vi "TDMS文件浏览.vi"() -> ()   [LabVIEW 2010]
doc: "Writes channels of data to different groups in the TDMS file format."
panel:
  in  "file path":path caption="文件路径"
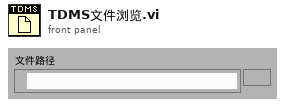
[diagram p1: front panel]
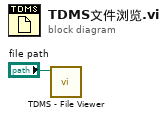
[diagram p0: block diagram]
diagram:
  n1 = call <vilib>:"TDMS - File Viewer.vi"("file path"="file path") -> ()  [unwired: 5 in, 2 out]
